vi "Configure Classic Monitor.vi"(8 "error in (no error)":errorcluster, 10 "Enable Orphan Detection? (T)":bool=TRUE) -> (0 "error out":errorcluster, 2 "Classic Monitor out":refnum<class "Actor Monitor.lvclass">)   [LabVIEW 2023, in "Monitored Actor.lvlib"]
doc: "Configures the Classic AF monitor window. Orphan Detection is enabled by default.\n\nPlease see the following web address for additional documentation and tutorial information:\nhttp://www.mooregoodideas.com/monitoring-actors/\n\nAuthor: Derek Trepanier\n\nCopyright (c) 2014, Moore Good Ideas, Inc.\n\nAll rights reserved.\n\nRedistribution and use in source and binary forms, with or without modification, are permitted provided that the following conditions are met:\n\n * Redistributions of source code must retain the above copyright notice, this list of conditions and the following disclaimer.\n * Redistributions in binary form must reproduce the above copyright notice, this list of conditions and the following disclaimer in the documentation and/or other materials provided with the distribution.\n * Neither the name of Moore Good Ideas, Inc. nor the names of its contributors may be used to endorse or promote products derived from this software without specific prior written permission.\n\nTHIS SOFTWARE IS PROVIDED BY THE COPYRIGHT HOLDERS AND CONTRIBUTORS \"AS IS\" AND ANY EXPRESS OR IMPLIED WARRANTIES, INCLUDING, BUT NOT LIMITED TO, THE IMPLIED WARRANTIES OF MERCHANTABILITY AND FITNESS FOR A PARTICULAR PURPOSE ARE DISCLAIMED. IN NO EVENT SHALL THE COPYRIGHT OWNER OR CONTRIBUTORS BE LIABLE FOR ANY DIRECT, INDIRECT, INCIDENTAL, SPECIAL, EXEMPLARY, OR CONSEQUENTIAL DAMAGES (INCLUDING, BUT NOT LIMITED TO, PROCUREMENT OF SUBSTITUTE GOODS OR SERVICES; LOSS OF USE, DATA, OR PROFITS; OR BUSINESS INTERRUPTION) HOWEVER CAUSED AND ON ANY THEORY OF LIABILITY, WHETHER IN CONTRACT, STRICT LIABILITY, OR TORT (INCLUDING NEGLIGENCE OR OTHERWISE) ARISING IN ANY WAY OUT OF THE USE OF THIS SOFTWARE, EVEN IF ADVISED OF THE POSSIBILITY OF SUCH DAMAGE."
uses:
  Library/Monitored Actor.lvlib
  Actor Monitor/Actor Monitor/Actor Monitor.lvclass
  Classic Monitor/Monitor/Monitor Actor/Classic Monitor.lvclass
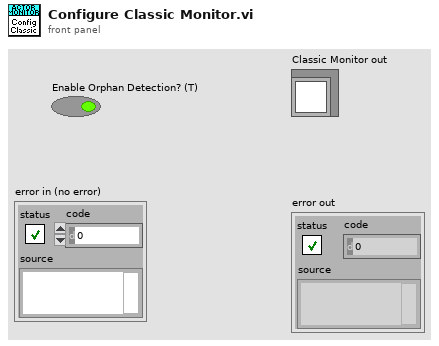
[diagram p1: front panel]
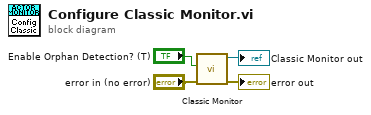
[diagram p0: block diagram]
diagram:
  n1 = call "Classic Monitor.vi"("error in (no error)"="error in (no error)", "Enable Orphan Detection?"="Enable Orphan Detection? (T)") -> ("error out"=→"error out":errorcluster, "Classic Monitor out"=→"Classic Monitor out":refnum<class "Classic Monitor.lvclass">)  [unwired: 8 in]
